vi "trace_properties_all.vi"(0 "reference in":refnum<class "OSA.lvclass">, 3 "dataType":T1, 5 "error in (no error)":errorcluster) -> (14 "reference out":refnum<class "OSA.lvclass">, 15 "properties":string[](array[string]), 17 "property values":string[][](array[string]), 19 "error out":errorcluster)   [LabVIEW 2010, in "OSA.lvclass"]
doc: "Trace properties returned as unsigned int, double and string arrays, (all)."
uses:
  OSA.lvclass
  typeDef/acq_dataType.ctl
  typeDef/trace_properties_string.ctl
  typeDef/trace_properties_ui.ctl
  typeDef/trace_properties_double.ctl
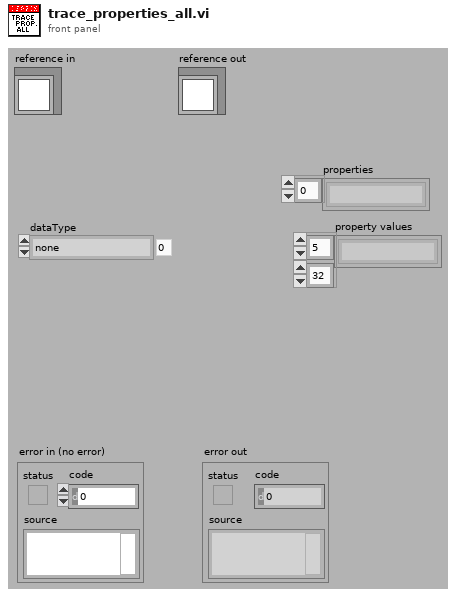
[diagram p1: front panel]
types:
  T1 = typedef "OSA.lvclass/acq_dataType.ctl" = enum16{"none", "interferogram", "spectrum"}
  T2 = typedef "OSA.lvclass/trace_properties_string.ctl" = enum16{"interferometerSerial [max 32]", "name [max 32]", "comment [max 128]", "source [max 24]", "instr_operator [max 24]", "instr_model_str [max 24]", "all_stringParameters"}
  T3 = typedef "OSA.lvclass/trace_properties_ui.ctl" = enum16{"length", "type", "acquisitionMode", "xValueFormat", "date", "time", "averageNum", "smoothType", "igramSmoothType", "phaseCorrection", "apodisation", "__allocatedLengthI", "__allocatedLengthx", "adcBits", "sensitivityMode", "resolutionMode", "rollingAverage", "samplesPerReference", "air_measureOption", "interferogramProperty", "all_uiProperties"}
  T4 = typedef "OSA.lvclass/trace_properties_double.ctl" = enum16{"x_minWnr", "x_maxWnr", "x_min", "x_max", "y_min", "y_max", "resolution", "referenceWavelength_nm_vac", "samplingDistance_cm_vac", "zeroFillFactor", "air_temp", "air_press", "air_relHum", "minOPD_cm", "maxOPD_cm", "interferogramOffset", "apodizationPowerCompensation", "integrationTime_ms", "gainLevel", "all_doubleProperties"}
  T5 = typedef "OSA.lvclass/ObjectAttributes.ctl" = cluster{"Stop":bool, "dataType":T1, "spectrometerIdx":u16, "buffer size interferogram":i32, "interferogram":cluster{"new":bool, "plot_x_ min":sgl, "plot_x_max":sgl, "plot_y_min":sgl, "plot_y_max":sgl, "Graph Intrfrgrm":T6, "timeStamp":u32, "signal (%)":dbl, "traces":cluster{"idx":u32, "broadBand":bool, "monoChromatic":bool, "peakToPeakSignal":dbl, "peakToPeakPos":dbl}[], "traces idx last":i32, "contrast (%)":dbl}, "spectrum":cluster{"new":bool, "plot_x_min":sgl, "plot_x_max":sgl, "plot_unit_x":T7, "plot_unit_y":T8, "plot_y_min":sgl, "plot_y_max":sgl, "Graph Spectrum":T6, "timeStamp":u32, "X_VAL_OPTIONS":enum16{"MIN_MAX", "ARRAY"}, "traces":cluster{"idx":u32}[], "traces idx last":i32}, "Thorlabs_OSA_64.lvclass:queue_action.ctlqueue ref":refnum<queue>, "action":T9, "plot zoom step":dbl, "buffer semaphore":T10, "acq stopped":bool, "dataType active":T1, "temperature (degr C)":sgl, "pressure (hPa)":sgl, "rel humidity (%)":sgl, "settings":cluster{"resolution":u16, "sensitivity":u16, "Average":bool, "average nr":u32, "apodisation":T11, "acq delay (ms)":u32, "airMesure":T12, "wmtr on":bool, "intfgrm_smooth_width":u16, "intfgrm_smooth_nrOfPasses":u16, "intfgrm_smooth":T13, "phaseCorrection":T14, "zeroFill":u8, "spectr_smooth":T13, "spectr_smooth_width":u16, "spectr_smooth_nrOfPasses":u16, "resolution (/cm)":sgl, "REF wavelength, (nm)":dbl, "gain_idx":u16, "gainAuto":bool, "gain_relative":dbl, "PD sensitivity mode":T15, "PD senseMode implemented":bool, "SensorTemperature implemented":bool, "SensorPressure implemented":bool, "SensorHumidity implemented":bool, "attenuationAuto":bool, "attenuationOnOff":bool, "attenuationAvailable":bool, "offsetAvailable":bool, "offset":i32, "offset max":u16, "contrastAvailable":bool}, "peaks position":sgl[], "peaks width":sgl[], "peaks height":sgl[], "peaks max nr":u32, "peaks latest nr":i32, "peaks new":bool, "power":dbl, "power new":bool, "path":string, "wavelength (WNr)":dbl, "wavelength new":bool, "buffer size spectrum":i32, "status":string, "vi reference":refnum<vi>, "funcPointer":u64, "libraryPointer":u64, "singleAcquisition":bool, "coherenceLength (cm)":dbl, "coherenceLength new":bool, "spectrometer model":string, "spectrometer serial nr":string, "peaks thld left":sgl[], "peaks thld right":sgl[], "coherenceLength error (cm)":dbl, "ADC bits":u16, "peaks position centroid":sgl[], "peaks height centroid":sgl[], "OSA series":T16, "channel index spectrum":u16, "spectrometer rangeLow, (/cm)":dbl, "spectrometer rangeHigh, (/cm)":dbl, "channel index interferogram":u16, "virtualSource":bool}
  T6 = typedef "OSA.lvclass/graph_intensity.ctl" = refnum<vi>
  T7 = typedef "OSA.lvclass/spectrum_x_unit.ctl" = enum16{"wavenr/cm", "THz", "eV", "nm_air", "nm_vac"}
  T8 = typedef "OSA.lvclass/y_unit.ctl" = enum16{"ADC counts", "dBm pwr absolute", "dBm pwr density", "mW pwr absolute", "mW pwr density"}
  T9 = typedef "OSA.lvclass/queue_action.ctl" = enum16{"none", "stop", "GUI_plotInterferogram", "GUI_plotSpectrum", "GUI_plotInterferogramRescale", "GUI_plotSpectrumRescale", "GUI_plotInterferogramReset", "GUI_plotSpectrumReset", "GUI_plotInterferogramAutoScaleY", "GUI_plotSpectrumAutoScaleY", "GUI_plotInterferogramZoomOut", "GUI_plotSpectrumZoomOut", "GUI_plotInterferogramPane", "GUI_plotSpectrumPane", "GUI_plotInterferogramZoomMouse", "GUI_plotSpectrumZoomMouse", "GUI_spectrumChannelType", "GUI_channel", "ENVIRONMENT temperature", "ENVIRONMENT pressure", "MODE_resolution set", "MODE_resolution get", "MODE_sensitivity set", "MODE_sensitivity get", "MODE_PDTemperature set", "MODE_PDTemperature get", "REBOOT/RESET firmware", "ACQASYNC_acquireSingleSpectrum", "ACQASYNC_continuous start", "ACQASYNC_continuous stop\n", "ACQASYNC_get last interferogram", "ACQASYNC_get last spectrum", "ACQASYNC_get last waveNr", "ACQOPT_interferogram smoothing set", "ACQOPT_interferogram smoothing get", "ACQOPT_spectrum smoothing set", "ACQOPT_spectrum smoothing get", "ACQOPT_apodisation type set", "ACQOPT_apodisation type get", "ACQOPT_phase correction type set", "ACQOPT_phase correction type get", "ACQOPT_acqIntervall_set", "ACQOPT_acqIntervall_get", "ACQOPT_average spectrum set", "ACQOPT_average spectrum get", "ACQOPT_rolling average set", "ACQOPT_rolling average get", "ACQOPT_zero fill factor set", "ACQOPT_zero fill factor get", "ACQOPT_cycle counting set", "ACQOPT_cycle counting get", "ACQOPT_air measure option set", "ACQOPT_air measure option get", "ACQOPT_gainLevel auto get", "ACQOPT_gainLevel auto set", "ACQOPT_gainLevel get", "ACQOPT_gainLevel set", "ACQOPT_offset set", "ACQOPT_attenuator_auto_set", "ACQOPT_attenuator_set", "ACQOPT_getAll", "INSTRUMENT_PROPERTY_range_WaveNr_min", "INSTRUMENT_PROPERTY_range_WaveNr_max", "INSTRUMENT_PROPERTY_reference_wavelength_cm^-1", "INSTRUMENT_PROPERTY_samplesPerRefPeriod", "INSTRUMENT_PROPERTY_resolution_waveNrPercm", "INSTRUMENT_PROPERTY_availableGainLevels", "INSTRUMENT_PROPERTY_status", "CONVERT", "ANALYSE_POWER", "ANALYSE_PEAKS", "ANALYSE_WAVELENGTH", "ANALYSE_SPECTRUM", "ANALYSE_INTERFEROGRAM", "ANALYSE_COHERENCE_LENGTH", "MATH", "MATH_power", "MATH_peaks", "FILE", "miscellaneous"}
  T10 = typedef "Semaphore RefNum" = refnum<k1>
  T11 = typedef "OSA.lvclass/apodisation.ctl" = enum16{"NONE", "NORTON_BEER_WEAK", "NORTON_BEER_MEDIUM", "NORTON_BEER_STRONG", "TRIANGULAR", "COSINE", "HANN", "HAMMING", "BLACKMANHARRIS3", "BLACKMANHARRIS4", "GAUSSIAN"}
  T12 = typedef "OSA.lvclass/airMeasure.ctl" = enum16{"TEMPERATURE", "PRESSURE"}
  T13 = typedef "OSA20X_misc.lvlib/interferogram_smoothing.ctl" = enum16{"NONE", "BINOMIAL", "SAVITSKY_GOLAY", "FOURIER", "MOVING_AVERAGE", "GAUSSIAN"}
  T14 = typedef "OSA.lvclass/phaseCorrection.ctl" = enum16{"NONE", "MERTZ", "FORMAN", "MERTZ_FILE", "FORMAN_FILE", "FUTURE COMP."}
  T15 = typedef "OSA20X_misc.lvlib/PDTemperatureMode.ctl" = enum16{"cool: better sensitivity/noise floor", "warm: extended wl range"}
  T16 = typedef "OSA.lvclass/OSA_series.ctl" = enum16{"OSA200", "OSA300", "UNKNOWN"}
  T17 = cluster{"idx":u32, "broadBand":bool, "monoChromatic":bool, "peakToPeakSignal":dbl, "peakToPeakPos":dbl}[]
  T18 = cluster{"property":string, "property value":string}[]
  T19 = cluster{"property":string, "property value":u32}[]
  T20 = cluster{"property":string, "property value":dbl}[]
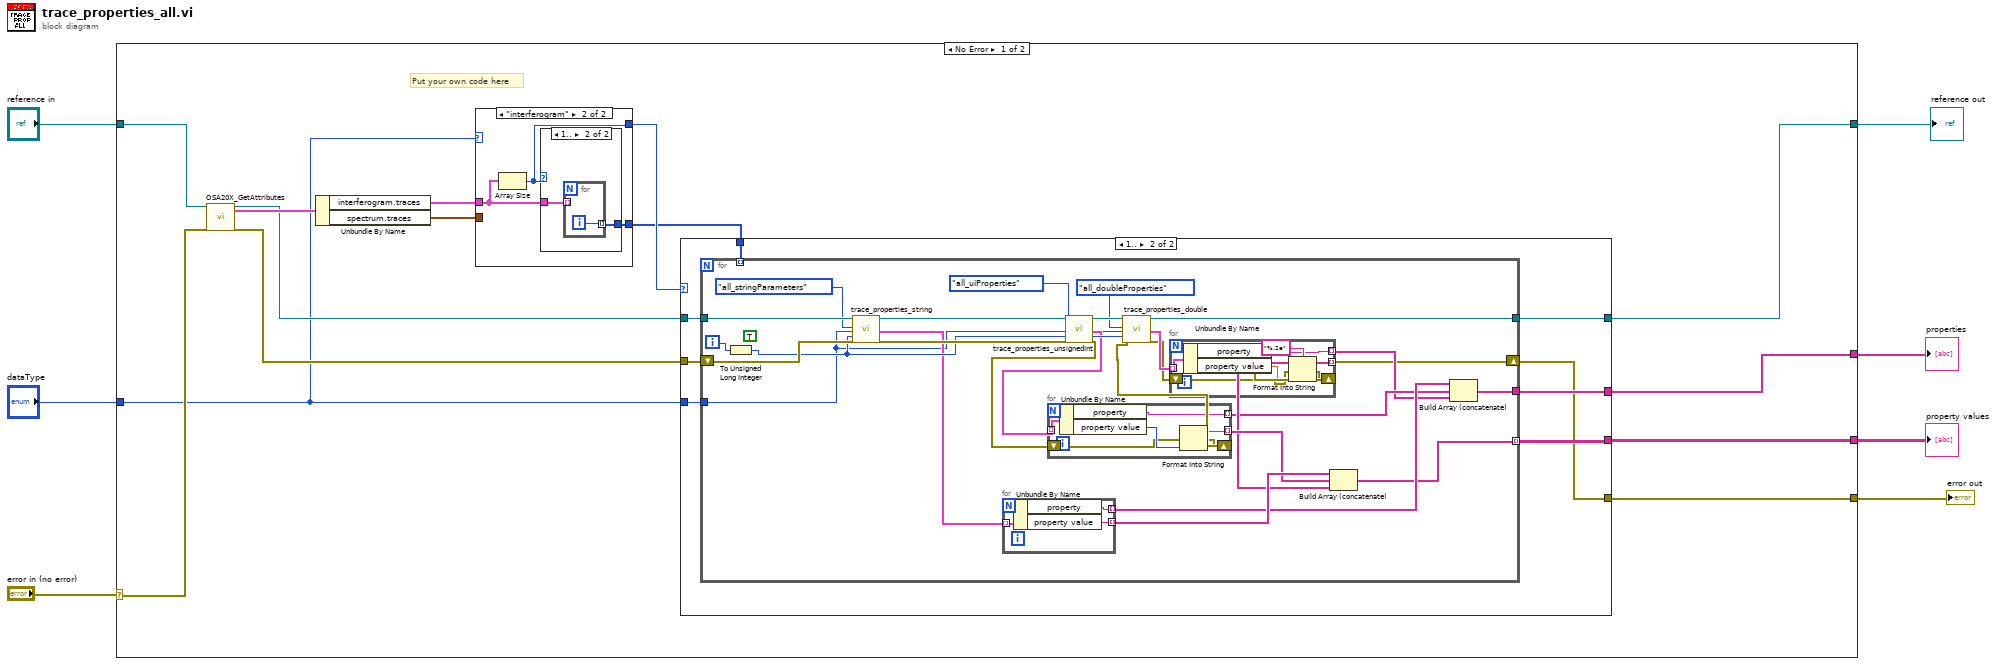
[diagram p0: block diagram]
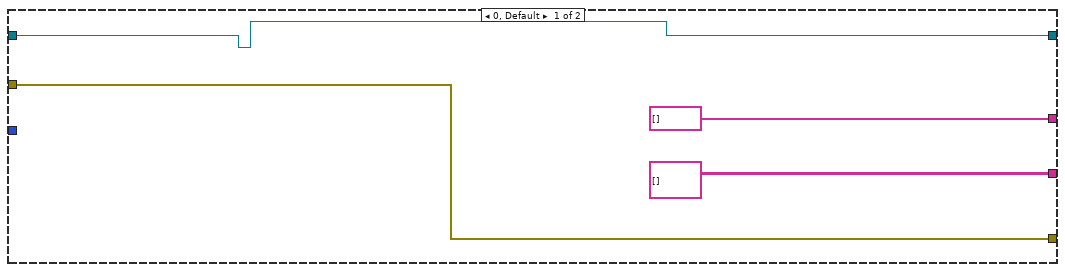
[diagram p2: hidden frame]
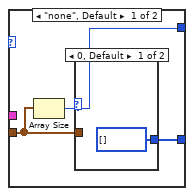
[diagram p3: hidden frame]
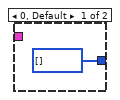
[diagram p5: hidden frame]
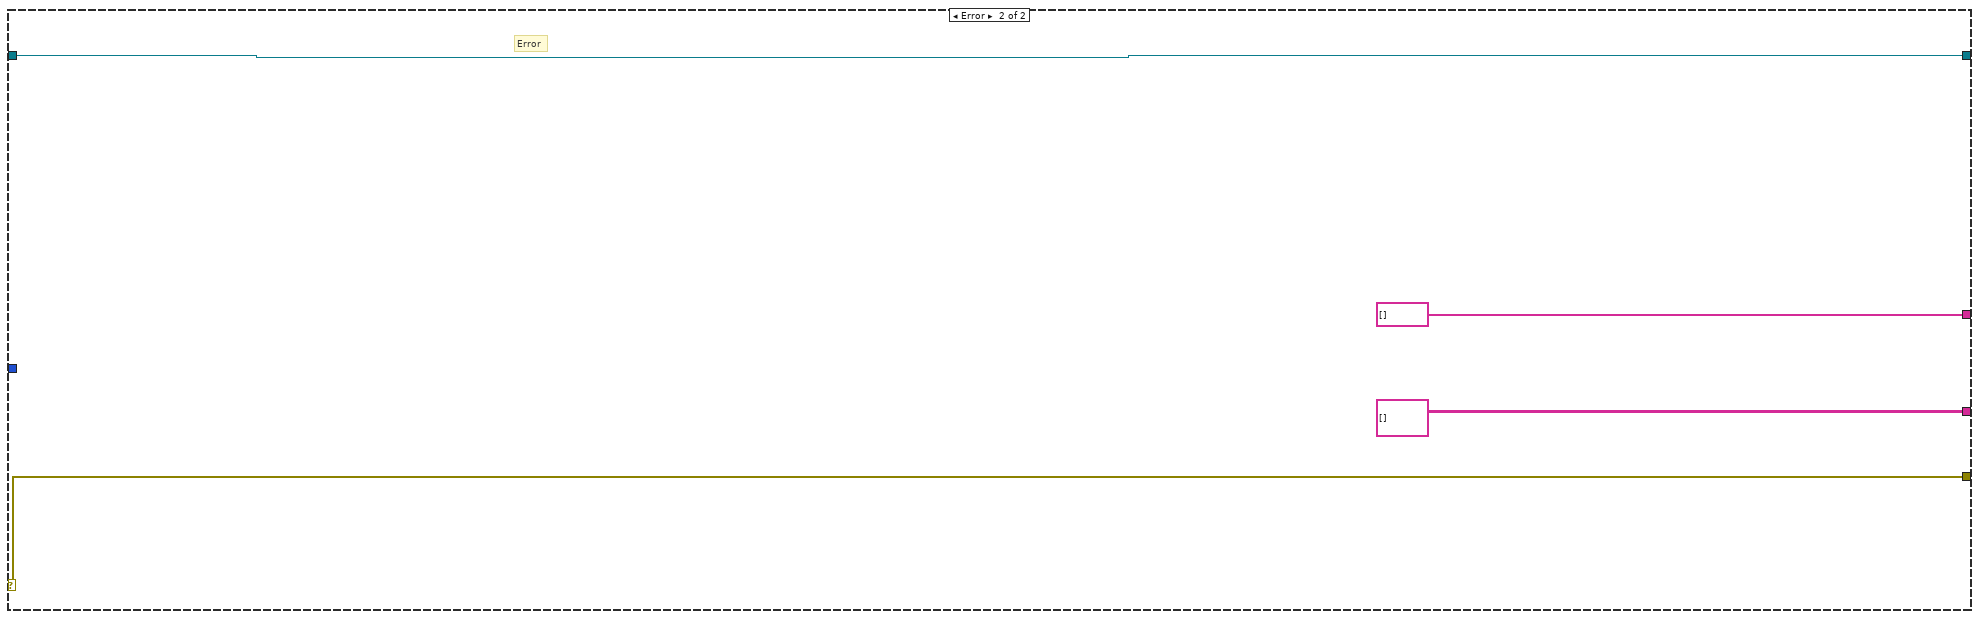
[diagram p6: hidden frame]
diagram:
  n1 = case shown="No Error" "error in (no error)" {
    selector: "error in (no error)" -> [w17 w94]
    tunnel: [w8 w94] -> w7
    tunnel: "reference in" -> [w18 w93]
    tunnel: [w16 w93] -> w4
    tunnel: "dataType" -> [w15 _]
    tunnel: [w10 string[] []] -> w2
    tunnel: [w9 string[][] []] -> w1
    frame No Error {
      # "Put your own code here"
      n2 = call "OSA20X_GetAttributes.vi"("reference in"=w18, "error in (no error)"=w17) -> ("reference out"=w19:refnum<class "OSA.lvclass">, "Data"=w21:T5, "error out"=w20:errorcluster)  [unwired: 14 in, 1 out]
      n3 = Unbundle By Name(w21) -> ("interferogram.traces"=w14:T17, "spectrum.traces"=w13:cluster{"idx":u32}[])
      n4 = case shown="\"interferogram\"" w15 {
        tunnel: w14 -> [_ w85]
        tunnel: w13 -> [w79 _]
        tunnel: [w78 w86] -> w12
        tunnel: [w77 w84] -> w11
        frame "none", Default {
          n5 = Array Size(array=w79) -> (size(s)=w78:i32)
          n6 = case shown="0, Default" w78 {
            tunnel: w79 -> [_ w81]
            tunnel: [i32[] [] w82] -> w77
            frame 0, Default {
            }
            frame 1.. {
              n7 = for {
                tunnel: [w83] -> w82 mode=indexing
                tunnel: w81 -> [_] mode=indexing
                i -> [w83]
              }
            }
          }
        }
        frame "interferogram" {
          n8 = Array Size(array=w85) -> (size(s)=w86:i32)
          n9 = case shown="1.." w86 {
            tunnel: w85 -> [_ w89]
            tunnel: [i32[] [] w88] -> w84
            frame 0, Default {
            }
            frame 1.. {
              n10 = for {
                tunnel: w89 -> [_] mode=indexing
                tunnel: [w90] -> w88 mode=indexing
                i -> [w90]
              }
            }
          }
        }
      }
      n11 = case shown="1.." w12 {
        tunnel: w20 -> [w25 w33]
        tunnel: w19 -> [w24 w27]
        tunnel: [w24 w26] -> w16
        tunnel: w15 -> [_ w32]
        tunnel: w11 -> [_ w31]
        tunnel: [string[] [] w30] -> w10
        tunnel: [string[][] [] w29] -> w9
        tunnel: [w25 w28] -> w8
        frame 0, Default {
        }
        frame 1.. {
          n12 = for {
            shift-right: [w40] -> w28
            shift-left: w33 -> [w59]
            tunnel: [w42] -> w29 mode=indexing
            tunnel: [w41] -> w30
            tunnel: w32 -> [w39]
            tunnel: w31 -> [_] mode=indexing
            tunnel: w27 -> [w37]
            tunnel: [w36] -> w26
            i -> [w35]
            (unwired) TRUE
            n13 = To Unsigned Long Integer(number=w35) -> (unsigned 32bit integer=w55:u32)
            n14 = call "trace_properties_string.vi"("reference in"=w37, "property"=trace_properties_string."all_stringParameters", "dataType"=w39, "trace idx"=w55, "error in (no error)"=w59) -> ("reference out"=w58:refnum<class "OSA.lvclass">, "property out array"=w54:T18, "error out"=w60:errorcluster)  [unwired: 11 in, 1 out]
            n15 = for {
              tunnel: w54 -> [w76] mode=indexing
              tunnel: [w75] -> w48 mode=indexing
              tunnel: [w74] -> w45 mode=indexing
              n16 = Unbundle By Name(w76) -> ("property"=w74:string, "property value"=w75:string)
            }
            n17 = call "trace_properties_unsignedInt.vi"("reference in"=w58, "property"=trace_properties_ui."all_uiProperties", "dataType"=w39, "trace idx"=w55, "error in (no error)"=w60) -> ("reference out"=w57:refnum<class "OSA.lvclass">, "property out array"=w53:T19, "error out"=w51:errorcluster)  [unwired: 10 in, 2 out]
            n18 = for {
              tunnel: w53 -> [w73] mode=indexing
              shift-right: [w70] -> w50
              shift-left: w51 -> [w71]
              tunnel: [w69] -> w47 mode=indexing
              tunnel: [w68] -> w44 mode=indexing
              n19 = Unbundle By Name(w73) -> ("property"=w68:string, "property value"=w72:u32)
              n20 = Format Into String(error in=w71, w72) -> (resulting string=w69:string, error out=w70:errorcluster)  [unwired: 2 in]
            }
            n21 = call "trace_properties_double.vi"("reference in"=w57, "property"=trace_properties_double."all_doubleProperties", "dataType"=w39, "trace idx"=w55, "error in (no error)"=w50) -> ("reference out"=w36:refnum<class "OSA.lvclass">, "property out array"=w52:T20, "error out"=w49:errorcluster)  [unwired: 11 in, 1 out]
            n22 = for {
              tunnel: w52 -> [w67] mode=indexing
              shift-right: [w64] -> w40
              shift-left: w49 -> [w63]
              tunnel: [w62] -> w46 mode=indexing
              tunnel: [w61] -> w43 mode=indexing
              n23 = Unbundle By Name(w67) -> ("property"=w61:string, "property value"=w66:dbl)
              n24 = Format Into String(format string="%.2e", error in=w63, w66) -> (resulting string=w62:string, error out=w64:errorcluster)  [unwired: 1 in]
            }
            n25 = Build Array (concatenate)(w48, w47, w46) -> (w42:string[])
            n26 = Build Array (concatenate)(w45, w44, w43) -> (w41:string[])
          }
        }
      }
    }
    frame Error {
      # "Error"
    }
  }
  "error out" <- w7
  "reference out" <- w4
  "properties" <- w2
  "property values" <- w1
